vi "historyLogPath.vi"(4 "error in":errorcluster) -> (0 "error out":errorcluster, 1 "Not a Path?":bool, 3 "Path Out":path)   [LabVIEW 2023]
uses:
  <vilib>/Utility/sysdir.llb/System Directory Type.ctl
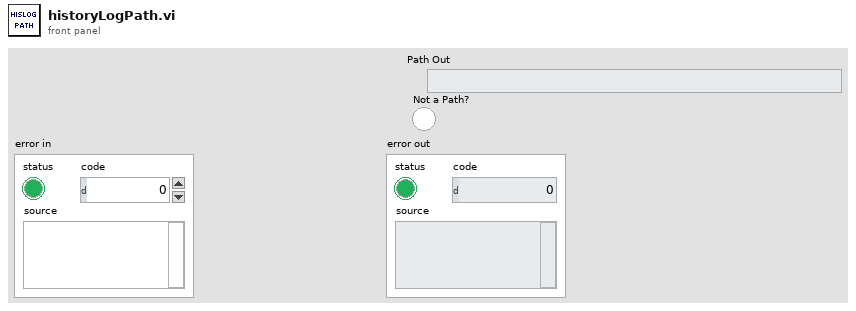
[diagram p1: front panel]
types:
  T1 = typedef "System Directory Type.ctl" = i32
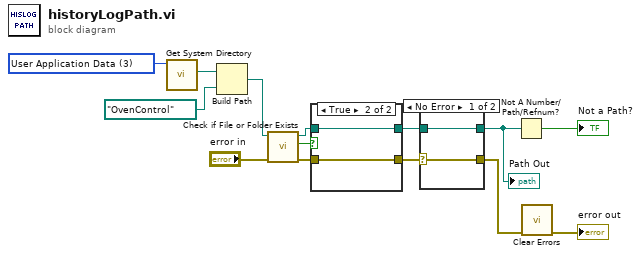
[diagram p0: block diagram]
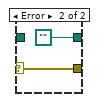
[diagram p2: hidden frame]
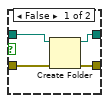
[diagram p3: hidden frame]
diagram:
  w14 = T1 3 items=["User Home"=0, "User Desktop"=1, "User Documents"=2, "User Application Data"=3, "User Preferences"=4, "User Temporary"=5, "Public Documents"=6, "Public Application Data"=7, "Public Preferences"=8, "Public Cache"=13, "System Core Libraries"=9, "System Installed Libraries"=10, "Application Files"=11, "Boot Volume Root"=12] ("system directory type")
  n1 = call <vilib>:"Get System Directory.vi"("system directory type"=w14) -> ("system directory"=w13:path)  [unwired: 10 in]
  n2 = Build Path(base path=w13, name or relative path=path "OvenControl") -> (appended path=w11:path)
  n3 = call <vilib>:"Check if File or Folder Exists.vi"("error in (no error)"="error in", "path"=w11) -> ("error out"=w7:errorcluster, "file or folder exists?"=w10:bool, "dup path"=w9:path)  [unwired: 7 in]
  n4 = case shown="True" w10 {
    tunnel: w9 -> [w18 w19]
    tunnel: w7 -> [w17 w20]
    tunnel: [w16 w20] -> w6
    tunnel: [w15 w19] -> w3
    frame False {
      n5 = Create Folder(path (use dialog)=w18, error in=w17) -> (created path=w15:path, error out=w16:errorcluster)  [unwired: 1 in, 1 out]
    }
    frame True {
    }
  }
  n6 = case shown="No Error" w6 {
    selector: w6 -> [w22 w24]
    tunnel: [w22 w24] -> w5
    tunnel: [w21 path ""] -> w2
    tunnel: w3 -> [w21 _]
    frame No Error {
    }
    frame Error {
    }
  }
  "Path Out" <- w2
  n7 = Not A Number/Path/Refnum?(number/path/refnum=w2) -> (NaN/Path/Refnum?=→"Not a Path?":bool)
  n8 = call <vilib>:"Clear Errors.vi"("error in (no error)"=w5) -> ("error out"=→"error out":errorcluster)  [unwired: 5 in, 1 out]
